vi "Start Monitor Helper.vi"(8 "error in (no error)":errorcluster, 11 "Lasers ON?":bool=TRUE) -> (0 "error out":errorcluster)   [LabVIEW 2015, in "Tool Module.lvlib"]
doc: "<b>Note:</b> This VI was modified by the <b>Validate DQMH Module</b> tool to turn off automatic error handling."
uses:
  Tool Module.lvlib
  _HS Data Stream Params Cluster--typedef.ctl
  _HS Data Stream SM enum--typedef.ctl
  Tool Interface/Tool Interface.lvlib
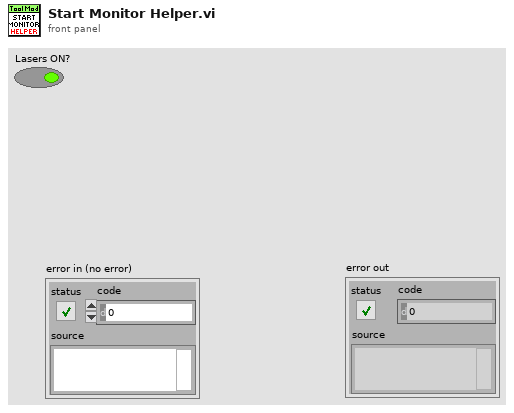
[diagram p1: front panel]
types:
  T1 = typedef "Tool Module.lvlib/_HS Data Stream SM enum--typedef.ctl" = enum16{"Idle", "Receive HS Data", "Close Connection"}
  T2 = typedef "Tool Module.lvlib/_HS Data Stream Params Cluster--typedef.ctl" = cluster{"Raw Data Stream Loop cmd":T1, "Data Array DVR ref":refnum<data-value>, "HS Sample Data notifier":refnum<notifier>, "Block Count Notifier":refnum<notifier>}
  T3 = typedef "Tool Module.lvlib/_Loop Ctrl Notifiers Cluster--typedef.ctl" = cluster{"Raw Stream Ctrl":refnum<notifier>}
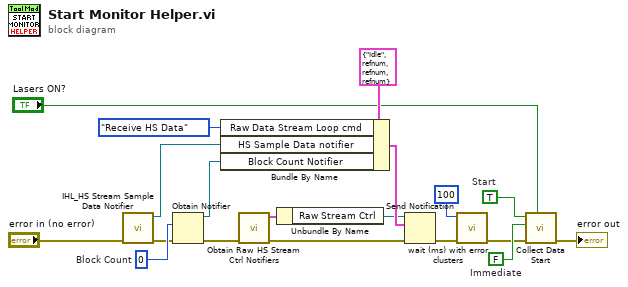
[diagram p0: block diagram]
diagram:
  w13 = FALSE  # Immediate
  w14 = TRUE  # Start
  w10 = u32 0  # Block Count
  n1 = call "IHL_HS Stream Sample Data Notifier.vi"("error in (no error)"="error in (no error)") -> ("error out"=w7:errorcluster, "Sample Data notifier out"=w19:refnum<notifier>)  [unwired: 9 in]
  n2 = Obtain Notifier(notification data type=w10, error in (no error)=w7) -> (notifier out=w6:refnum<notifier>, error out=w15:errorcluster)  [unwired: 2 in, 1 out]
  n3 = Bundle By Name(cluster=T2 {"Raw Data Stream Loop cmd"=enum."Idle", "Data Array DVR ref"=refnum, "HS Sample Data notifier"=refnum, "Block Count Notifier"=refnum} ("_HS Data Stream Params Cluster--typedef"), "Raw Data Stream Loop cmd"=_HS_Data_Stream_SM_enum--typedef."Receive HS Data" ("HS Data Stream SM enum"), "HS Sample Data notifier"=w19, "Block Count Notifier"=w6) -> (w12:T2)
  n4 = call "Obtain Raw HS Stream Ctrl Notifiers.vi"("error in (no error)"=w15) -> ("error out"=w11:errorcluster, "Loop Ctrl Notifiers Cluster"=w8:T3)  [unwired: 9 in]
  n5 = Unbundle By Name(w8) -> ("Raw Stream Ctrl"=w9:refnum<notifier>)
  n6 = Send Notification(notification=w12, notifier=w9, error in (no error)=w11) -> (error out=w17:errorcluster)  [unwired: 1 out]
  n7 = call "wait (ms) with error clusters.vi"("error in (no error)"=w17, "milliseconds to wait"=u32 100 ("milliseconds")) -> ("error out"=w4:errorcluster)  [unwired: 9 in]
  n8 = call "Collect Data Start.vi"("Lasers ON?"="Lasers ON?", "error in (no error)"=w4, "Immediate"=w13, "Start"=w14) -> ("error out"=→"error out":errorcluster)  [unwired: 7 in]
